vi "rosbridge_read.vi"(8 "error in (no error)":errorcluster, 10 "stop":bool, 11 "TCP Network Connection in":refnum<k5>) -> (0 "error out":errorcluster, 2 "String":string, 3 "TCP Network Connection out":refnum<k5>)   [LabVIEW 2013]
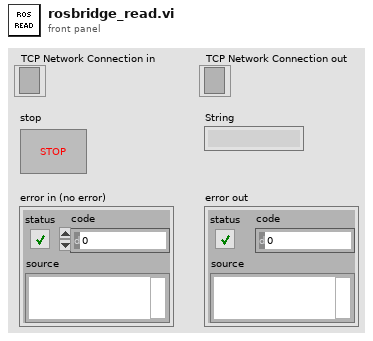
[diagram p1: front panel]
types:
  T1 = enum16{"Standard", "Buffered", "CRLF", "Immediate"}
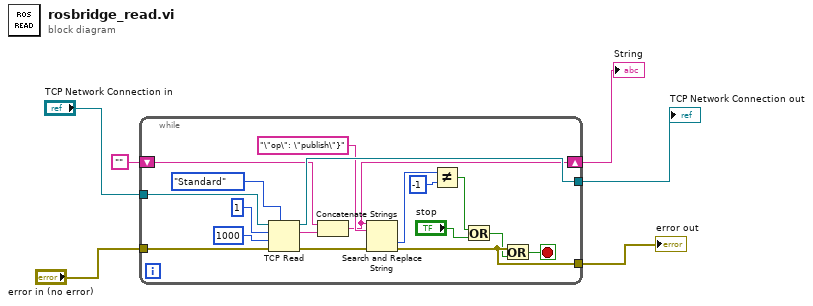
[diagram p0: block diagram]
diagram:
  n1 = while {
    tunnel: [w22] -> w1
    tunnel: [w15] -> w5
    tunnel: "TCP Network Connection in" -> [w23]
    tunnel: "error in (no error)" -> [w18]
    shift-right: [w8] -> w6
    shift-left: "" -> [w10]
    stop <- w24 stop-if-true
    n2 = TCP Read(connection ID=w23, bytes to read=1, error in (no error)=w18, 7:T1."Standard" ("mode (standard)"), 9:1000 ("timeout ms (25000)")) -> (connection ID out=w22:refnum<k5>, data out=w9:string, error out=w16:errorcluster)
    n3 = Concatenate Strings(w10, w9) -> (w8:string)
    n4 = Search and Replace String(input string=w8, search string="\"op\": \"publish\"}", error in=w16) -> (offset past replacement=w12:i32, error out=w15:errorcluster)  [unwired: 5 in, 2 out]
    n5 = Not Equal?(x=w12, y=-1) -> (x != y?=w14:bool)
    n6 = Or(x=w14, y="stop") -> (x .or. y?=w11:bool)
    n7 = Or(x=w15, y=w11) -> (x .or. y?=w24:bool)
  }
  "String" <- w6
  "error out" <- w5
  "TCP Network Connection out" <- w1
